vi "Get DI Camera Info.vi"(8 "error in (no error)":errorcluster, 11 "info":u32) -> (0 "error out":errorcluster, 2 "function return":u32, 3 "info out":u32)   [LabVIEW 2014, in "atmcd32d.lvlib"]
doc: "unsigned int WINAPI GetDICameraInfo(void * info);"
uses:
  atmcd32d.lvlib
  atmcd32d.dll
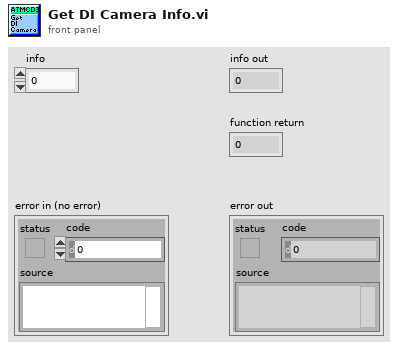
[diagram p1: front panel]
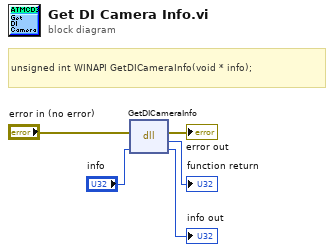
[diagram p0: block diagram]
diagram:
  # "unsigned int WINAPI GetDICameraInfo(void * info);"
  n1 = dll-call lib="C:/Users/Bakir/Documents/Lambda2-Testing/lib/Andorlib/atmcd32d.*" fn="GetDICameraInfo"(error in="error in (no error)", "info"="info") -> (error out=→"error out":errorcluster, →"function return":u32, "info"=→"info out":u32)  [unwired: 2 in, 1 out]
